vi "Load.vi"(8 "error in":errorcluster, 10 "Source":string="D:\\git\\HAL\\Source\\Tests\\resources\\instruments.xlsx", 11 "Config from Excel Table in":refnum<class "Config from Excel Table.lvclass">) -> (0 "error out":errorcluster, 3 "Config from Excel Table out":refnum<class "Config from Excel Table.lvclass">)   [LabVIEW 2025, in "Config from Excel Table.lvclass"]
uses:
  Config from Excel Table.lvclass
  Config from Excel Table.lvclass/Config from Excel Table.ctl
  <vilib>/Peter/Open Xml/Source/Open Xml.lvlib
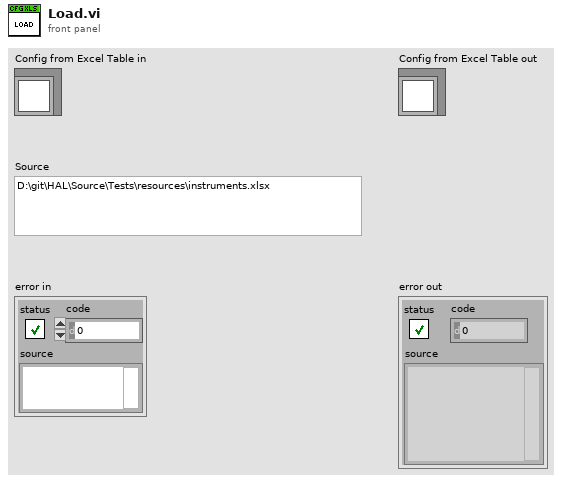
[diagram p1: front panel]
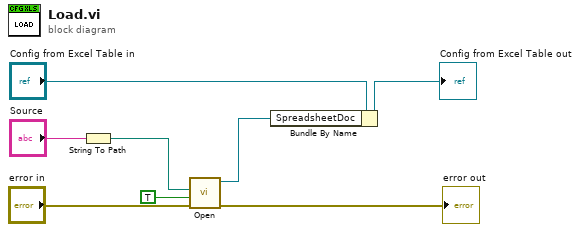
[diagram p0: block diagram]
diagram:
  n1 = String To Path(string="Source") -> (path=w1:path)
  n2 = call <vilib>:"Open.vi"("error in"="error in", "isEditable"=TRUE, "Path"=w1) -> ("error out"=→"error out":errorcluster, "SpreadsheetDoc"=w2:refnum<k24>)  [unwired: 7 in]
  n3 = Bundle By Name(cluster="Config from Excel Table in", "SpreadsheetDoc"=w2) -> (→"Config from Excel Table out":refnum<class "Config from Excel Table.lvclass">)
